vi "Set Current Iteration.vi"(8 "error in (no error)":errorcluster, 10 "iteration":u64=1, 11 "Transfer Group in":refnum<class "Transfer Group.lvclass">) -> (0 "error out":errorcluster, 3 "Transfer Group out":refnum<class "Transfer Group.lvclass">)   [LabVIEW 2017, in "DSF Core.lvlib" / "Transfer Group.lvclass"]
uses:
  Transfer Group.lvclass
  Transfer Group.lvclass/Transfer Group.ctl
  Timing/Timing.lvclass/Timing.ctl
  Timing/Set Iteration.vi
  Timing/Timing.lvclass
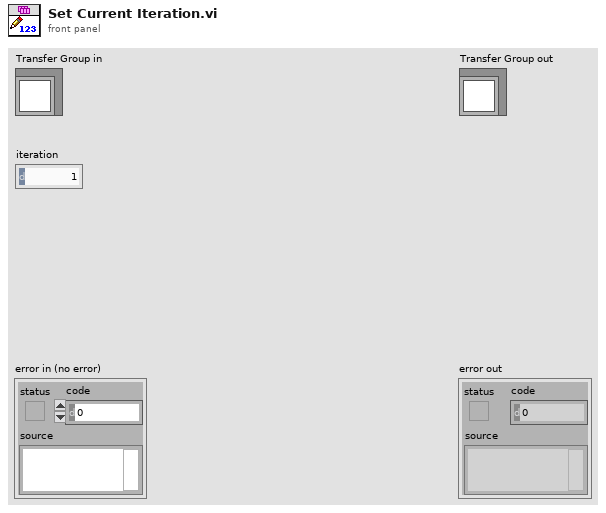
[diagram p1: front panel]
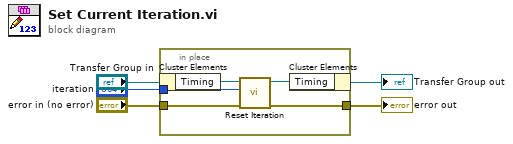
[diagram p0: block diagram]
diagram:
  n1 = in-place {
    in-place-border: "error in (no error)" -> [w10]
    in-place-border: [w9] -> w4
    in-place-border: "iteration" -> [w8]
    n2 = in-place-cluster #1("Transfer Group in") -> ("Timing"=w7:refnum<class "Timing.lvclass">)
    n3 = call "Reset Iteration.vi"("error in (no error)"=w10, "iteration"=w8, "Timing in"=w7) -> ("error out"=w9:errorcluster, "Timing out"=w6:refnum<class "Timing.lvclass">)  [unwired: 7 in]
    n4 = in-place-cluster #1("Timing"=w6) -> (→"Transfer Group out":refnum<class "Transfer Group.lvclass">)
  }
  "error out" <- w4
